vi "GetLastError.vi"(11 "error in (no error)":errorcluster) -> (4 "pErrorCode":i32, 6 "pszErrText":string, 8 "pSize":u64, 10 "GX_STATUS":i32, 15 "error out":errorcluster)   [LabVIEW 2016, in "GxLVLib.lvlib"]
uses:
  GxLVLib.lvlib
  GxIAPI.dll
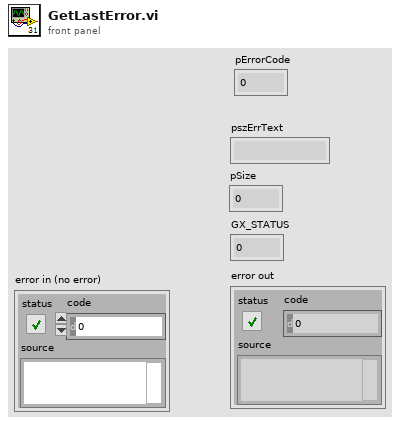
[diagram p1: front panel]
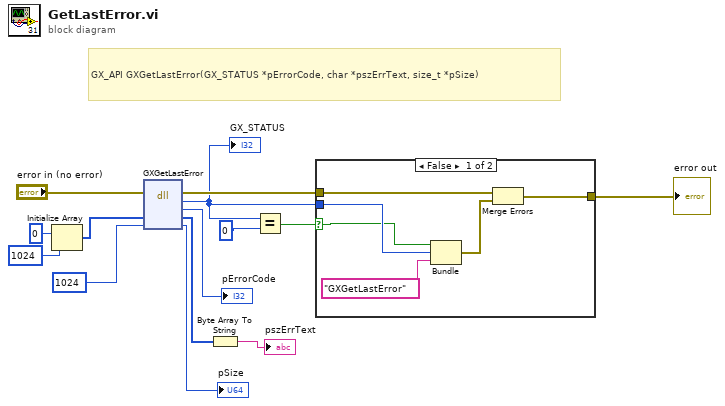
[diagram p0: block diagram]
diagram:
  # "GX_API GXGetLastError(GX_STATUS *pErrorCode, char *pszErrText, size_t *pSize)"
  n1 = Initialize Array(i8 0 ("element"), 1024 ("dimension size")) -> (w4:i8[])
  n2 = dll-call lib="GxIAPI.dll" fn="GXGetLastError"(error in="error in (no error)", "pszErrText"=w4, "pSize"=u64 1024) -> (error out=w12:errorcluster, "GX_STATUS"=w9:i32, "pErrorCode"=→"pErrorCode":i32, "pszErrText"=w7:i8[], "pSize"=→"pSize":u64)  [unwired: 3 in, 1 out]
  "GX_STATUS" <- w9
  n3 = Byte Array To String(unsigned byte array=w7) -> (string=→"pszErrText":string)
  n4 = Equal?(x=w9, y=0) -> (x = y?=w11:bool)
  n5 = case shown="False" w11 {
    selector: w11 -> [w16 _]
    tunnel: w12 -> [w20 w21]
    tunnel: [w19 w21] -> w13
    tunnel: w9 -> [w17 _]
    frame False {
      n6 = Bundle(w16, "GX_STATUS"=w17, "GXGetLastError") -> (w18:cluster{bool, "GX_STATUS":i32, string})  [unwired: 1 in]
      n7 = Merge Errors(w20, w18) -> (w19:errorcluster)
    }
    frame True {
    }
  }
  "error out" <- w13
